vi "Validate User Credentials.vi"(0 "User Configuration Manager in":refnum<class "User Configuration Manager.lvclass">, 5 "Username":string, 7 "Password":string, 11 "error in (no error)":errorcluster) -> (4 "User Configuration Manager out":refnum<class "User Configuration Manager.lvclass">, 6 "User Found":bool, 8 "Verified":bool, 10 "Verification Message":string, 15 "error out":errorcluster)   [LabVIEW 2017, in "User Configuration Manager.lvlib" / "User Configuration Manager.lvclass"]
doc: "Verifies the credentials of the user specified by user name."
uses:
  User Configuration Manager.lvclass
  User Configuration Manager.lvclass/User Configuration Manager.ctl
  140db478-7e3e-4888-bb9f-0cf7b5b1b4d2.vi
  Accessors/Read Linked List Ref .vi
  Read Encryption Type.vi
  <vilib>/gpm_packages/@cs/linked-list/Source/Linked List/ILinkedList/ILinked List.lvclass
  iEncryption/iEncryption.lvclass
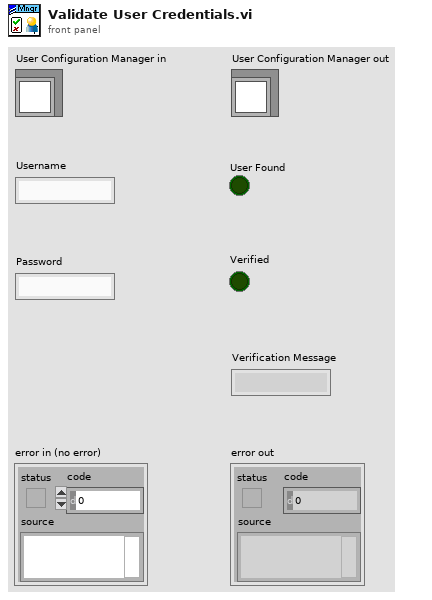
[diagram p1: front panel]
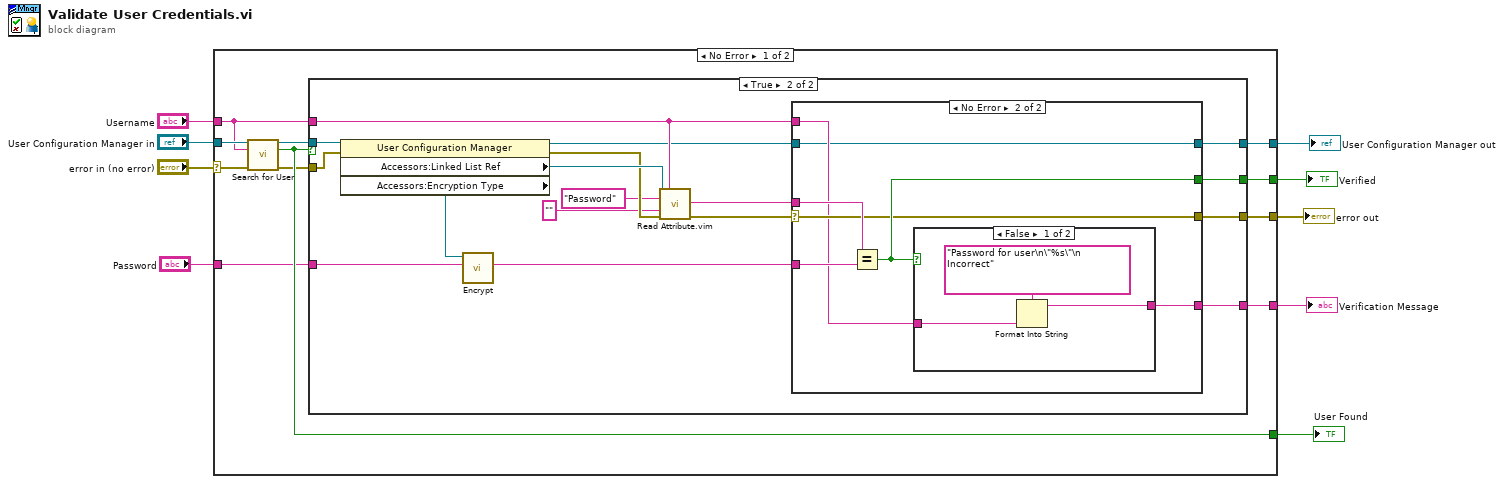
[diagram p0: block diagram]
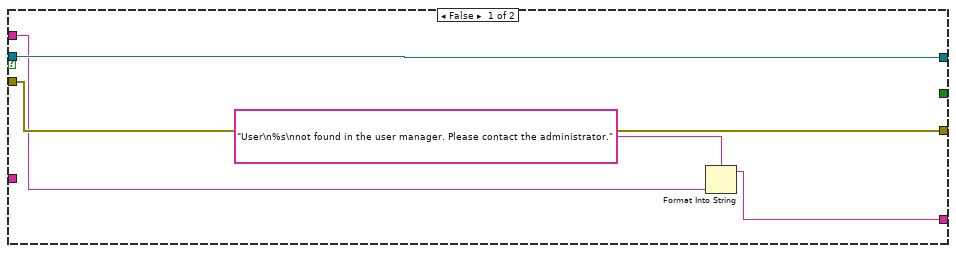
[diagram p2: hidden frame]
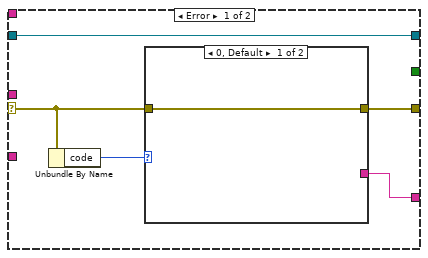
[diagram p3: hidden frame]
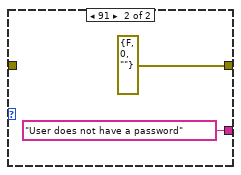
[diagram p4: hidden frame]
diagram:
  n1 = case shown="No Error" "error in (no error)" {
    selector: "error in (no error)" -> [w19 w61]
    tunnel: "User Configuration Manager in" -> [w20 w62]
    tunnel: "Password" -> [w14 _]
    tunnel: "Username" -> [w15 _]
    tunnel: [w11 w62] -> w7
    tunnel: [w10 w61] -> w6
    tunnel: [w12 _] -> w3
    tunnel: [w13 _] -> w2
    tunnel: [w17 _] -> w1
    frame No Error {
      n2 = call-dynamic "Search for User.vi"("User Configuration Manager in"=w20, "Username"=w15, "error in (no error)"=w19) -> ("User Configuration Manager out"=w18:refnum<class "User Configuration Manager.lvclass">, "Found"=w17:bool, "error out"=w16:errorcluster)  [unwired: 10 in]
      n3 = case shown="True" w17 {
        tunnel: w18 -> [w24 w42]
        tunnel: w16 -> [w25 w40]
        tunnel: w15 -> [w21 w31]
        tunnel: w14 -> [_ w29]
        tunnel: [w22 w35] -> w13
        tunnel: [_ w33] -> w12
        tunnel: [w24 w26] -> w11
        tunnel: [w25 w32] -> w10
        frame False {
          n4 = Format Into String(format string="User\n%s\nnot found in the user manager. Please contact the administrator.", w21) -> (resulting string=w22:string)  [unwired: 2 in, 1 out]
        }
        frame True {
          n5 = property class="User Configuration Manager"(reference=w42, error in=w40) -> (reference out=w27:refnum<class "User Configuration Manager.lvclass">, error out=w39:errorcluster, "Accessors:Linked List Ref "=w41:refnum<data-value>, "Accessors:Encryption Type"=w30:refnum<class "iEncryption.lvclass">)
          n6 = call-dynamic "Encrypt.vi"("String"=w29, "iEncryption in"=w30) -> ("Encrypted String"=w28:string)  [unwired: 9 in]
          n7 = call "Read Attribute.vim"("Linked List Ref"=w41, "Linked List ID"=w31, "Attribute Name"="Password", "Type"="" ("Attribute Name"), "error in (no error)"=w39) -> ("Attribute"=w36:string, "error out"=w34:errorcluster)  [unwired: 5 in, 4 out]
          n8 = case shown="No Error" w34 {
            selector: w34 -> [w44 w54]
            tunnel: w36 -> [_ w57]
            tunnel: w28 -> [_ w56]
            tunnel: [w47 w52] -> w35
            tunnel: [_ w55] -> w33
            tunnel: [w46 w54] -> w32
            tunnel: w31 -> [_ w53]
            tunnel: [w43 w51] -> w26
            tunnel: w27 -> [w43 w51]
            frame Error {
              n9 = Unbundle By Name(w44) -> ("code"=w45:i32)
              n10 = case shown="0, Default" w45 {
                tunnel: [_ "User does not have a password"] -> w47
                tunnel: [w48 errorcluster {"status"=FALSE, "code"=0, "source"=""} ("error out")] -> w46
                tunnel: w44 -> [w48 _]
                frame 0, Default {
                }
                frame 91 {
                }
              }
            }
            frame No Error {
              n11 = Equal?(x=w57, y=w56) -> (x = y?=w55:bool)
              n12 = case shown="False" w55 {
                tunnel: w53 -> [w59 _]
                tunnel: [w58 _] -> w52
                frame False {
                  n13 = Format Into String(format string="Password for user\n\"%s\"\n Incorrect", w59) -> (resulting string=w58:string)  [unwired: 2 in, 1 out]
                }
                frame True {
                }
              }
            }
          }
        }
      }
    }
    frame Error {
    }
  }
  "error out" <- w6
  "User Configuration Manager out" <- w7
  "Verified" <- w3
  "Verification Message" <- w2
  "User Found" <- w1
